vi "CryoServer Generate Ch Name Map.vi"() -> (3 "Generate Table":string[][](array[string]))   [LabVIEW 2021]
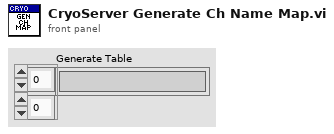
[diagram p1: front panel]
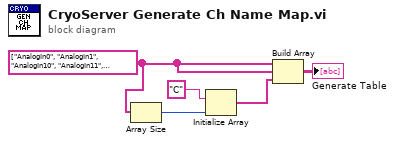
[diagram p0: block diagram]
diagram:
  w5 = string[] ["AnalogIn0", "AnalogIn1", "AnalogIn10", "AnalogIn11", "AnalogIn12", "AnalogIn2", "AnalogIn3", "AnalogIn4", "AnalogIn5", "AnalogIn6", "AnalogIn7", "AnalogIn8", "AnalogIn9", "Channel 0", "Channel 1", "Channel 10", "Channel 11", "Channel 12", "Channel 13", "Channel 14", "Channel 15", "Channel 2", "Channel 3", "Channel 4", "Channel 5", "Channel 6", "Channel 7", "Channel 8", "Channel 9", "aDac"] ("Ch Names")
  n1 = Array Size(array=w5) -> (size(s)=w4:i32)
  n2 = Initialize Array("C", w4) -> (w2:string[])
  n3 = Build Array(w5, w5, w2) -> (→"Generate Table":string[][])
